vi "Estrazione fondo Host Test RT.vi"() -> ()   [LabVIEW 2014]
uses:
  <vilib>/FPGAPlugInAG/sbRIO-9636/niLvFpga_Open_sbRIO-9636.vi
  <vilib>/rvi/interface/common/dynamic/niFpgaDynamicAddResources.vi
  <vilib>/Utility/error.llb/Error Cluster From Error Code.vi
  <vilib>/rvi/errors/niLvFpgaAdjustHostInterfaceError.vi
  <vilib>/rvi/interface/common/niFpgaWaitOnOcc.vi
  <vilib>/FPGAPlugInAG/Dynamic/niLvFpga_Run_Dynamic.vi
  <vilib>/FPGAPlugInAG/Dynamic/niLvFpga_Reset_Dynamic.vi
  <vilib>/FPGAPlugInAG/Dynamic/niLvFpga_Abort_Dynamic.vi
  <vilib>/rvi/interface/nirviOpenFPGA/nirviOpenFPGA.xnode
  FPGA Bitfiles/LaserDistanceSen_FPGATarget_EstrazioneFondo-_j5tEHZ7DPrM.lvbitx
  FPGA Target/Support VIs/Estrazione Fondo - Target.vi
  <vilib>/rvi/interface/nirviReadWriteControl/nirviReadWriteControl.xnode
  <vilib>/rvi/interface/nirviMethod/nirviMethod.xnode
  <vilib>/FPGAPlugInAG/Dynamic/niLvFpga_ConfigureFifo_Dynamic.vi
  <vilib>/rvi/errors/niLvFpgaMergeErrorWithErrorCode.vi
  <vilib>/FPGAPlugInAG/Dynamic/niLvFpga_StartFifo_Dynamic.vi
  NiFpgaLv.dll
  <vilib>/rvi/interface/Simulation/niFpgaSimulationCallBeginRW.vi
panel:
  out "Subtracted signal":dbl[](graph)
  in  "SubtractionType":T1(ring)
  out "Fondo Signal":dbl[](graph)
  out "Complete Mean Signal":dbl[](graph)
  in  "LowPass Filter: Low cutoff frequency":dbl=100000.0 format="%#_13g"
  in  "PolyFitting: Poly Grade":dbl=10.0
  in  "nbit":i32=8
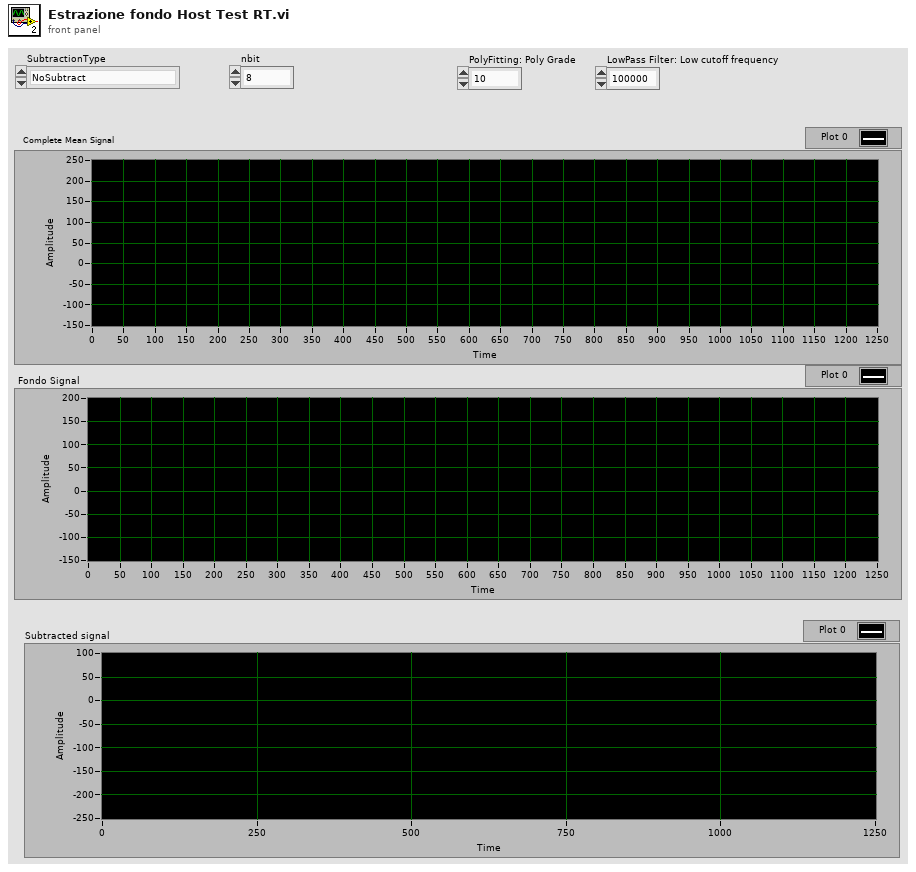
[diagram p1: front panel]
types:
  T1 = enum16{"NoSubtract", "StartingCurve", "LowPass", "PolyFitting"}
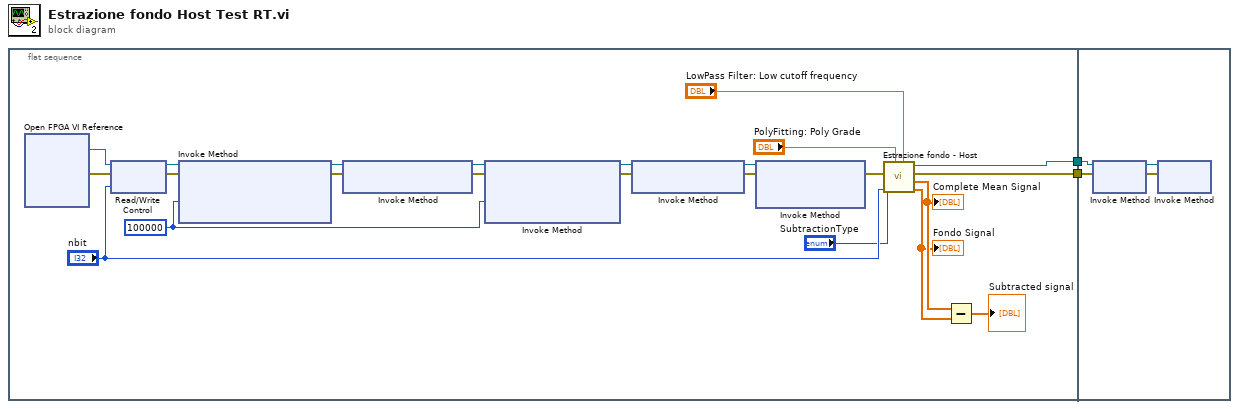
[diagram p0: block diagram]
diagram:
  n1 = flat-sequence {
    tunnel: [w11] -> w2
    tunnel: [w10] -> w1
    tunnel: w2 -> [w26]
    tunnel: w1 -> [w27]
    frame #0 {
      w23 = u32 100000 ("Requested Depth")
      n2 = xnode "Open FPGA VI Reference"() -> ("FPGA VI Reference Out"=w14:refnum<k20>, "error out"=w16:errorcluster)  [unwired: 2 in]
      n3 = xnode "Read/Write Control"("FPGA VI Reference In"=w14, "error in"=w16, "N-Mean"="nbit") -> ("FPGA VI Reference Out"=w13:refnum<k20>, "error out"=w15:errorcluster)
      n4 = xnode "Invoke Method"("FPGA VI Reference In"=w13, "error in"=w15, "Requested Depth"=w23) -> ("FPGA VI Reference Out"=w22:refnum<k20>, "error out"=w21:errorcluster)  [unwired: 1 out]
      n5 = xnode "Invoke Method"("FPGA VI Reference In"=w22, "error in"=w21) -> ("FPGA VI Reference Out"=w20:refnum<k20>, "error out"=w19:errorcluster)
      n6 = xnode "Invoke Method"("FPGA VI Reference In"=w20, "error in"=w19, "Requested Depth"=w23) -> ("FPGA VI Reference Out"=w25:refnum<k20>, "error out"=w24:errorcluster)  [unwired: 1 out]
      n7 = xnode "Invoke Method"("FPGA VI Reference In"=w25, "error in"=w24) -> ("FPGA VI Reference Out"=w18:refnum<k20>, "error out"=w17:errorcluster)
      n8 = xnode "Invoke Method"("FPGA VI Reference In"=w18, "error in"=w17) -> ("error out"=w12:errorcluster)  [unwired: 1 in, 1 out]
      n9 = call "Estrazione fondo - Host.vi"("LowPass Filter: Low cutoff frequency"="LowPass Filter: Low cutoff frequency", "PolyFitting: Poly Grade"="PolyFitting: Poly Grade", "nbit"="nbit", "SubtractionType"="SubtractionType", "error in"=w12) -> ("Fondo Signal"=w4:dbl[], "Complete Mean Signal"=w5:dbl[], "error out"=w11:errorcluster, "FPGA VI Reference Out"=w10:refnum<k20>)  [unwired: 3 in]
      "Complete Mean Signal" <- w5
      "Fondo Signal" <- w4
      n10 = Subtract(x=w5, y=w4) -> (x-y=→"Subtracted signal":dbl[])
    }
    frame #1 {
      n11 = xnode "Invoke Method"("FPGA VI Reference In"=w27, "error in"=w26) -> ("FPGA VI Reference Out"=w29:refnum<k20>, "error out"=w28:errorcluster)
      n12 = xnode "Invoke Method"("FPGA VI Reference In"=w29, "error in"=w28) -> ()  [unwired: 2 out]
    }
  }
